vi "1motorVelCtrl (SubVI).vi"(6 "reset Encoder":bool, 7 "Motor ID":T1, 8 "error in (no error)":errorcluster, 10 "motorSpeed (deg/s)":dbl(slide) scale=-450.0..450.0, 11 "TitanQuad in":refnum<class "TitanQuad.lvclass">) -> (0 "error out":errorcluster, 1 "Cluster":cluster{"Target (deg)":dbl, "Enc (deg)":dbl}, 2 "Enc (deg)":dbl, 3 "TitanQuad out":refnum<class "TitanQuad.lvclass">)   [LabVIEW 2020]
uses:
  <vilib>/CISH Robotics/L4VMX TitanQuad/Motor ID.ctl
  <vilib>/CISH Robotics/L4VMX TitanQuad/TitanQuad.lvclass
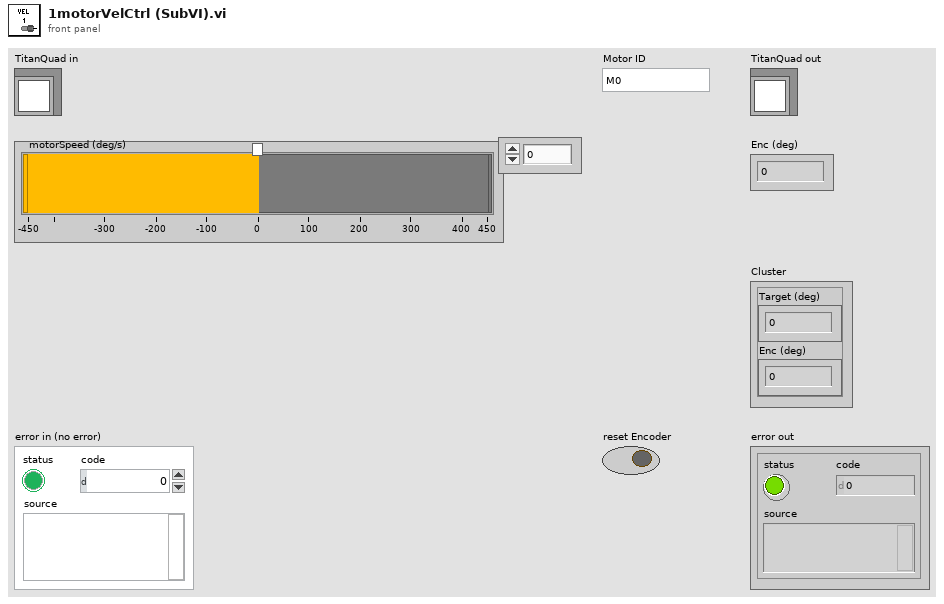
[diagram p1: front panel]
types:
  T1 = typedef "TitanQuad.lvlib/TitanQuad.lvclass/Motor ID.ctl" = enum16{"M0", "M1", "M2", "M3"}
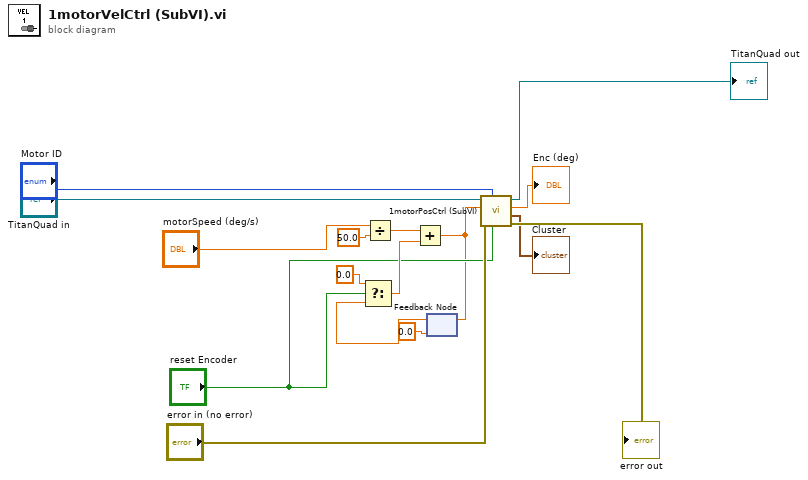
[diagram p0: block diagram]
diagram:
  n1 = Divide(x="motorSpeed (deg/s)", y=50.0) -> (x/y=w8:dbl)
  n2 = feedback #1(0.0) -> (w13:dbl)
  n3 = Select(t=0.0, s="reset Encoder", f=w13) -> (s? t:f=w14:dbl)
  n4 = Add(x=w8, y=w14) -> (x+y=w10:dbl)
  n5 = feedback-in #1(w10) -> ()
  n6 = call "1motorPosCtrl (SubVI).vi"("reset Encoder"="reset Encoder", "Motor ID"="Motor ID", "Error In"="error in (no error)", "Target (deg)"=w10, "TitanQuad in"="TitanQuad in") -> ("error out"=→"error out":errorcluster, "Cluster"=→"Cluster":cluster{"Target (deg)":dbl, "Enc (deg)":dbl}, "Enc (deg)"=→"Enc (deg)":dbl, "TitanQuad out"=→"TitanQuad out":refnum<class "TitanQuad.lvclass">)  [unwired: 3 in]
